vi "RT_stage_control_sine_following_Rev3.vi"() -> ()   [LabVIEW 2019]
uses:
  <vilib>/Platform/TimedLoop/XDataNode/timing_clust.ctl
  <vilib>/Platform/TimedLoop/XDataNode/nitl_modes.ctl
  <vilib>/Platform/TimedLoop/XDataNode/wakeup.ctl
  <vilib>/FPGAPlugInAG/myRIO-1900/niLvFpga_Open_myRIO-1900.vi
  <vilib>/rvi/interface/common/dynamic/niFpgaDynamicAddResources.vi
  <vilib>/Utility/error.llb/Error Cluster From Error Code.vi
  <vilib>/rvi/errors/niLvFpgaAdjustHostInterfaceError.vi
  <vilib>/rvi/interface/nirviOpenFPGA/nirviOpenFPGA.xnode
  FPGA Bitfiles/studentchallenge_FPGATarget_FPGARADCWDAC3_gNVwU-DQYMc.lvbitx
  FPGA_R_ADC_W_DAC.vi
  <vilib>/Platform/TimedLoop/XDataNode/XDataNode.xnode
  <vilib>/rvi/interface/nirviReadWriteControl/nirviReadWriteControl.xnode
  <vilib>/Platform/TimedLoop/XDataNode/XDNodeRunTimeDep.lvlib
  NiFpgaLv.dll
  <vilib>/rvi/interface/Simulation/niFpgaSimulationCallBeginRW.vi
panel:
  in  "Amplitude":dbl
  in  "Frequency":dbl
  in  "Offset":dbl
  out "N late finishes":i32
  out "Finished Late? [i-1]":bool
  in  "manual":dbl=-0.8009999999999999 step=0.03 format="%_6g"
  in  "PID control":bool
  in  "stop":bool
  in  "Reset Sensors":bool
  out "Displacement (mm)":cluster{"num refs":i16, dbl, "Y":dbl}(graph)
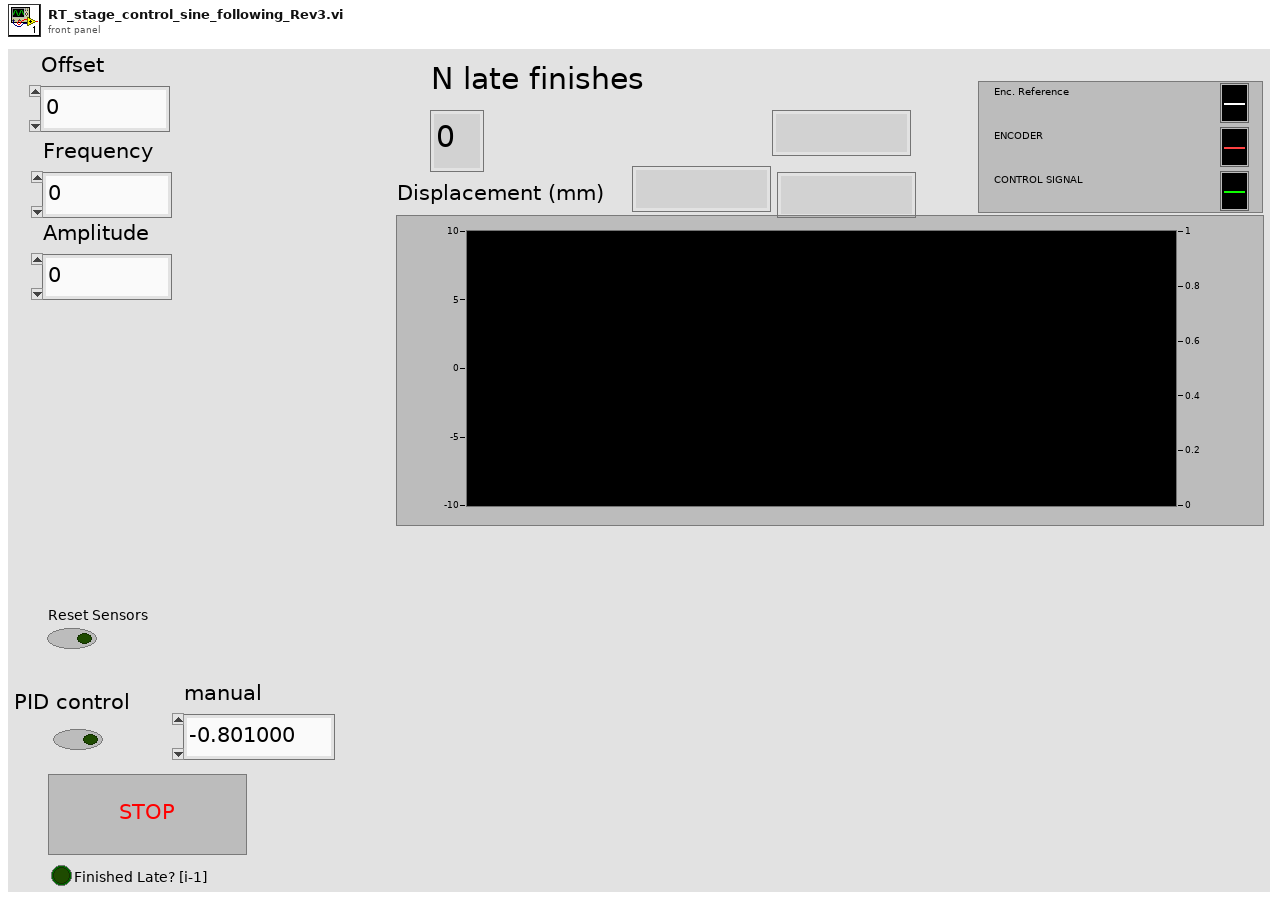
[diagram p1: front panel]
types:
  T1 = typedef "XDNodeRunTimeDep.lvlib/timing_clust.ctl" = cluster{"Expected End [f-1]":u64, "Actual End [f-1]":u64, "Finished Late? [f-1]":bool, "Expected End [i-1]":u64, "Actual End [i-1]":u64, "Finished Late? [i-1]":bool, "Expected Start [i]":u64, "Actual Start [i]":u64, "Expected Start [f]":u64, "Actual Start [f]":u64, "Source Name":string, "Structure Name":string, "Period":i64, "Deadline":i64, "Offset":i64, "Start":i64, "Priority":i32, "Timeout":i32, "Mode":T2, "Wakeup Reason":T3, "Error":errorcluster, "Source Type":string, "Secondary Source Type":string, "Global End Time":u64, "Global Start Time":u64, "Frame Duration":u64, "Iteration Duration":u64, "Assigned CPU":i32, "I/O Scan Engine Mode":u32}
  T2 = typedef "XDNodeRunTimeDep.lvlib/nitl_modes.ctl" = enum32{"No Change", "Process missed periods, maintain original phase", "Discard missed periods, maintain original phase", "Process missed periods, ignore original phase", "Discard missed periods, ignore original phase"}
  T3 = typedef "XDNodeRunTimeDep.lvlib/wakeup.ctl" = enum32{"Normal", "Aborted", "Asynchronous wakeup", "Timing source error", "Timed loop error", "Timeout"}
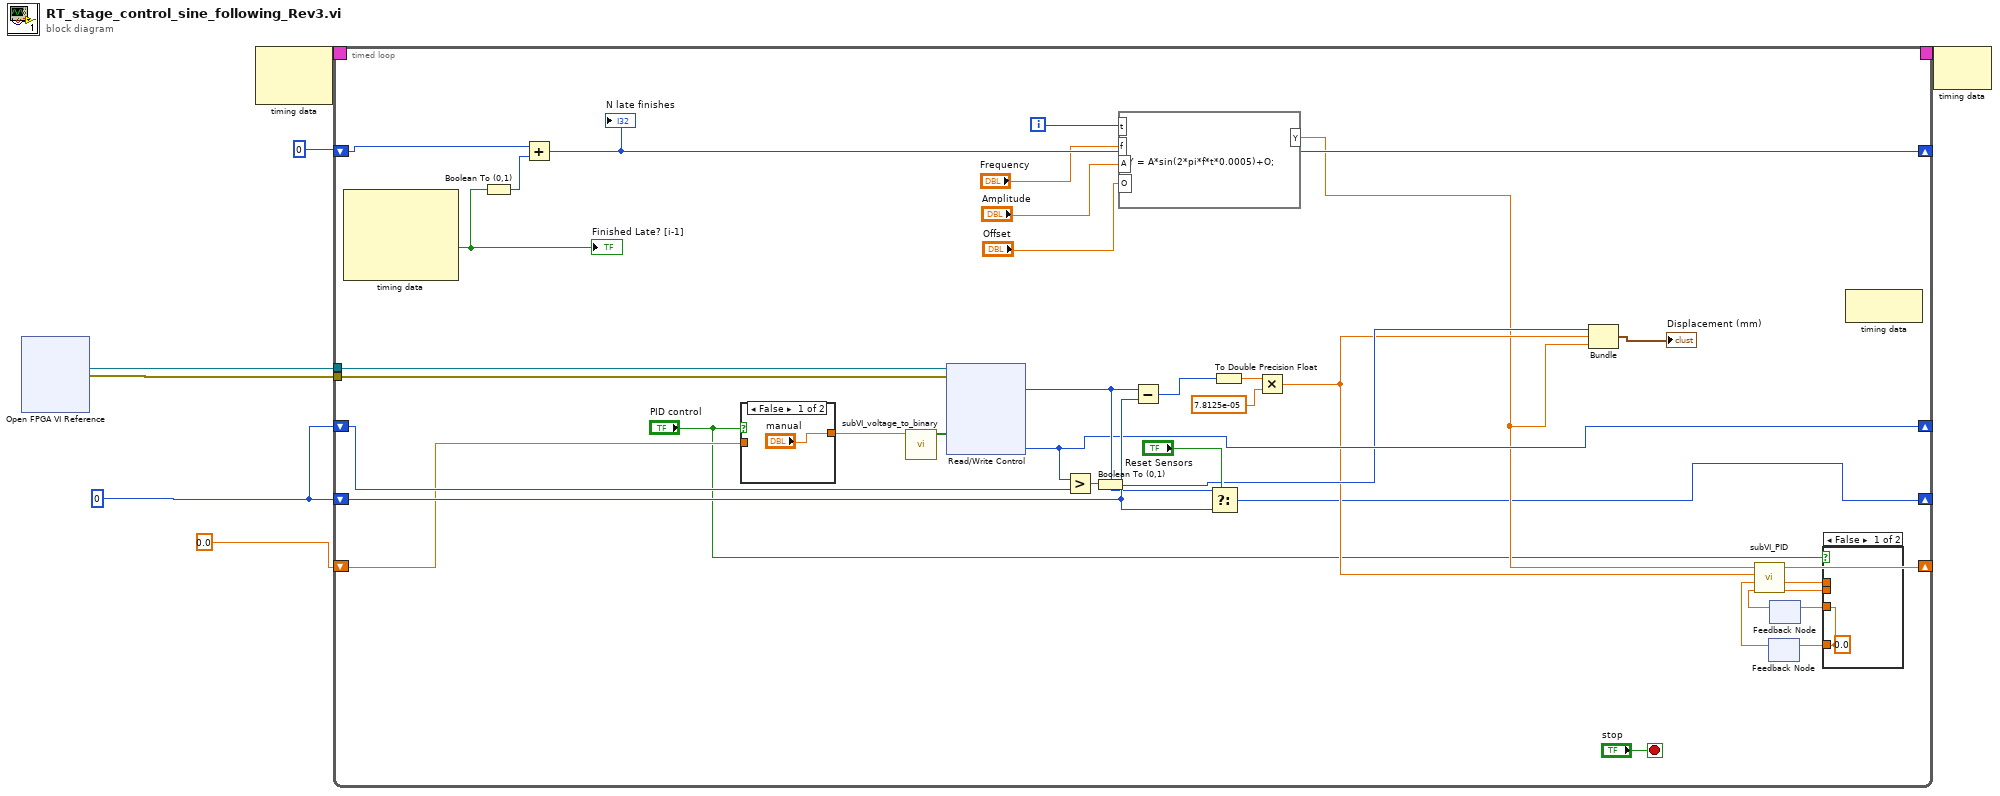
[diagram p0: block diagram]
diagram:
  w2 = 0
  n1 = xnode "Open FPGA VI Reference"() -> ("FPGA VI Reference Out"=w7:refnum<k20>, "error out"=w6:errorcluster)  [unwired: 2 in]
  n2 = node-c288() -> (w5:T1)  [unwired: 2 in]
  n3 = timed-loop {
    tunnel: w7 -> [w43]
    shift-right: [w15] -> _
    shift-left: w2 -> [w39]
    tunnel: w6 -> [w37]
    shift-right: [w18] -> _
    shift-left: 0.0 -> [w19]
    timing: w5 -> [_]
    timing-out: [_] -> w4
    shift-right: [w29] -> _
    shift-left: 0 -> [w30]
    shift-right: [w24] -> _
    shift-left: w2 -> [w23]
    i -> [w25]
    stop <- "stop" stop-if-true
    n4 = node-c288() -> (w32:bool)  [unwired: 1 in, 4 out]
    "Finished Late? [i-1]" <- w32
    n5 = Boolean To (0,1)(Boolean=w32) -> (0, 1=w31:i16)
    n6 = Add(x=w30, y=w31) -> (x+y=w29:i32)
    "N late finishes" <- w29
    n7 = case shown="False" "PID control" {
      tunnel: ["manual" w48] -> w34
      tunnel: w19 -> [_ w48]
      frame False {
      }
      frame True {
      }
    }
    n8 = call "subVI_voltage_to_binary.vi"("voltage"=w34) -> ("binary"=w38:bool[])  [unwired: 10 in]
    n9 = xnode "Read/Write Control"("FPGA VI Reference In"=w43, "error in"=w37, "DAC 1 write"=w38) -> ("Encoder A"=w35:i32, "num refs"=w24:i16)  [unwired: 1 in, 3 out]
    n10 = Greater?(x=w24, y=w23) -> (0:w22:bool)
    n11 = Boolean To (0,1)(Boolean=w22) -> (0, 1=w21:i16)
    n12 = formula code="Y = A*sin(2*pi*f*t*0.0005)+O;"("A"="Amplitude", "f"="Frequency", "t"=w25, "O"="Offset") -> ("Y"=w16:dbl)
    n13 = Subtract(x=w35, y=w39) -> (x-y=w40:i32)
    n14 = Select(t=w35, s="Reset Sensors", f=w39) -> (s? t:f=w15:i32)
    n15 = To Double Precision Float(number=w40) -> (double precision float=w41:dbl)
    n16 = Multiply(x=w41, y=7.8125e-05) -> (x*y=w17:dbl)
    n17 = Bundle(w21, w17, "Y"=w16) -> (→"Displacement (mm)":cluster{i16, dbl, "Y":dbl})  [unwired: 1 in]
    n18 = feedback #1() -> (w13:dbl)  [unwired: 1 in]
    n19 = feedback #2() -> (w14:dbl)  [unwired: 1 in]
    n20 = call "subVI_PID.vi"("Cumulative Error In"=w14, "Previous Error"=w13, "Encoder Position [mm]"=w17, "Desired Position [mm]"=w16) -> ("Cumulative Error Out"=w10:dbl, "Error"=w11:dbl, "Control Signal [V]"=w18:dbl)  [unwired: 5 in]
    n21 = case shown="False" "PID control" {
      tunnel: [w44 w46] -> w12
      tunnel: w11 -> [_ w46]
      tunnel: w10 -> [_ w45]
      tunnel: [w44 w45] -> w9
      frame False {
        w44 = 0.0 ("Error")
      }
      frame True {
      }
    }
    n22 = feedback-in #1(w12) -> ()
    n23 = feedback-in #2(w9) -> ()
    n24 = node-c288() -> ()  [unwired: 1 in, 1 out]
  }
  n25 = node-c288(w4) -> ()  [unwired: 1 out]
